vi "Release Queue.vi"(8 "error in (no error)":errorcluster, 11 "Queue in":refnum<class "Queue.lvclass">) -> (0 "error out":errorcluster, 3 "Queue out":refnum<class "Queue.lvclass">)   [LabVIEW 2012, in "Architecture.lvlib" / "Queue.lvclass"]
uses:
  Queue.lvclass
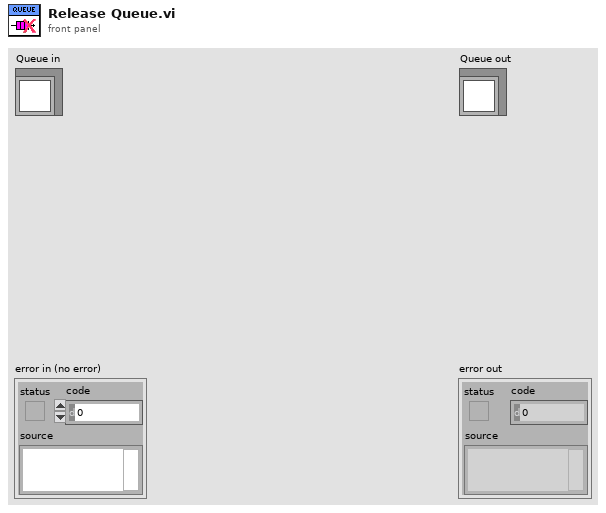
[diagram p1: front panel]
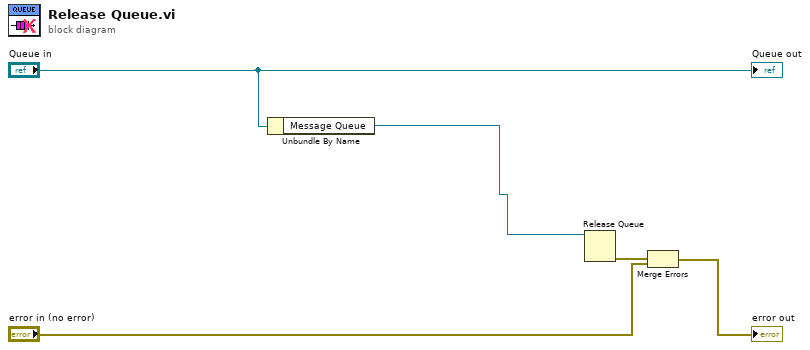
[diagram p0: block diagram]
diagram:
  n1 = Unbundle By Name("Queue in") -> ("Message Queue"=w2:refnum<queue>)
  n2 = Release Queue(queue=w2) -> (error out=w1:errorcluster)  [unwired: 2 in, 2 out]
  n3 = Merge Errors(w1, "error in (no error)") -> (→"error out":errorcluster)
  "Queue out" <- "Queue in"
